vi "Controller VI.vi"(6 "Current Time In":u32, 7 "Read String":string, 8 "Down Detect Time In":u32, 9 "Up Detect Time In":u32, 10 "Left Detect Time In":u32, 11 "Right Detect Time In":u32) -> (0 "Down Detect Time Out":u32, 1 "Up Detect Time Out":u32, 2 "Left Detect Time Out":u32, 3 "Right detect Time Out":u32, 4 "Control Cluster":T1 {"Yaw Speed" scale=-1.0..1.0; "Vertical Speed" scale=-1.0..1.0; "Pitch" scale=-1.0..1.0; "Roll" scale=-1.0..1.0}, 5 "Command string":string)   [LabVIEW 2014]
uses:
  Others/Control cluster.ctl
  Global.vi
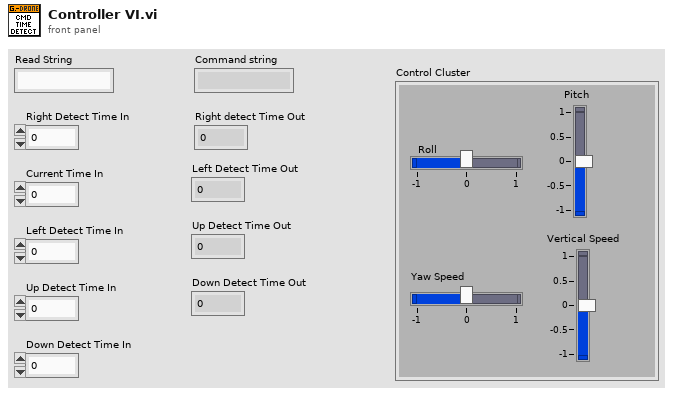
[diagram p1: front panel]
types:
  T1 = typedef "Control cluster.ctl" = cluster{"Roll":sgl, "Pitch":sgl, "Vertical Speed":sgl, "Yaw Speed":sgl}
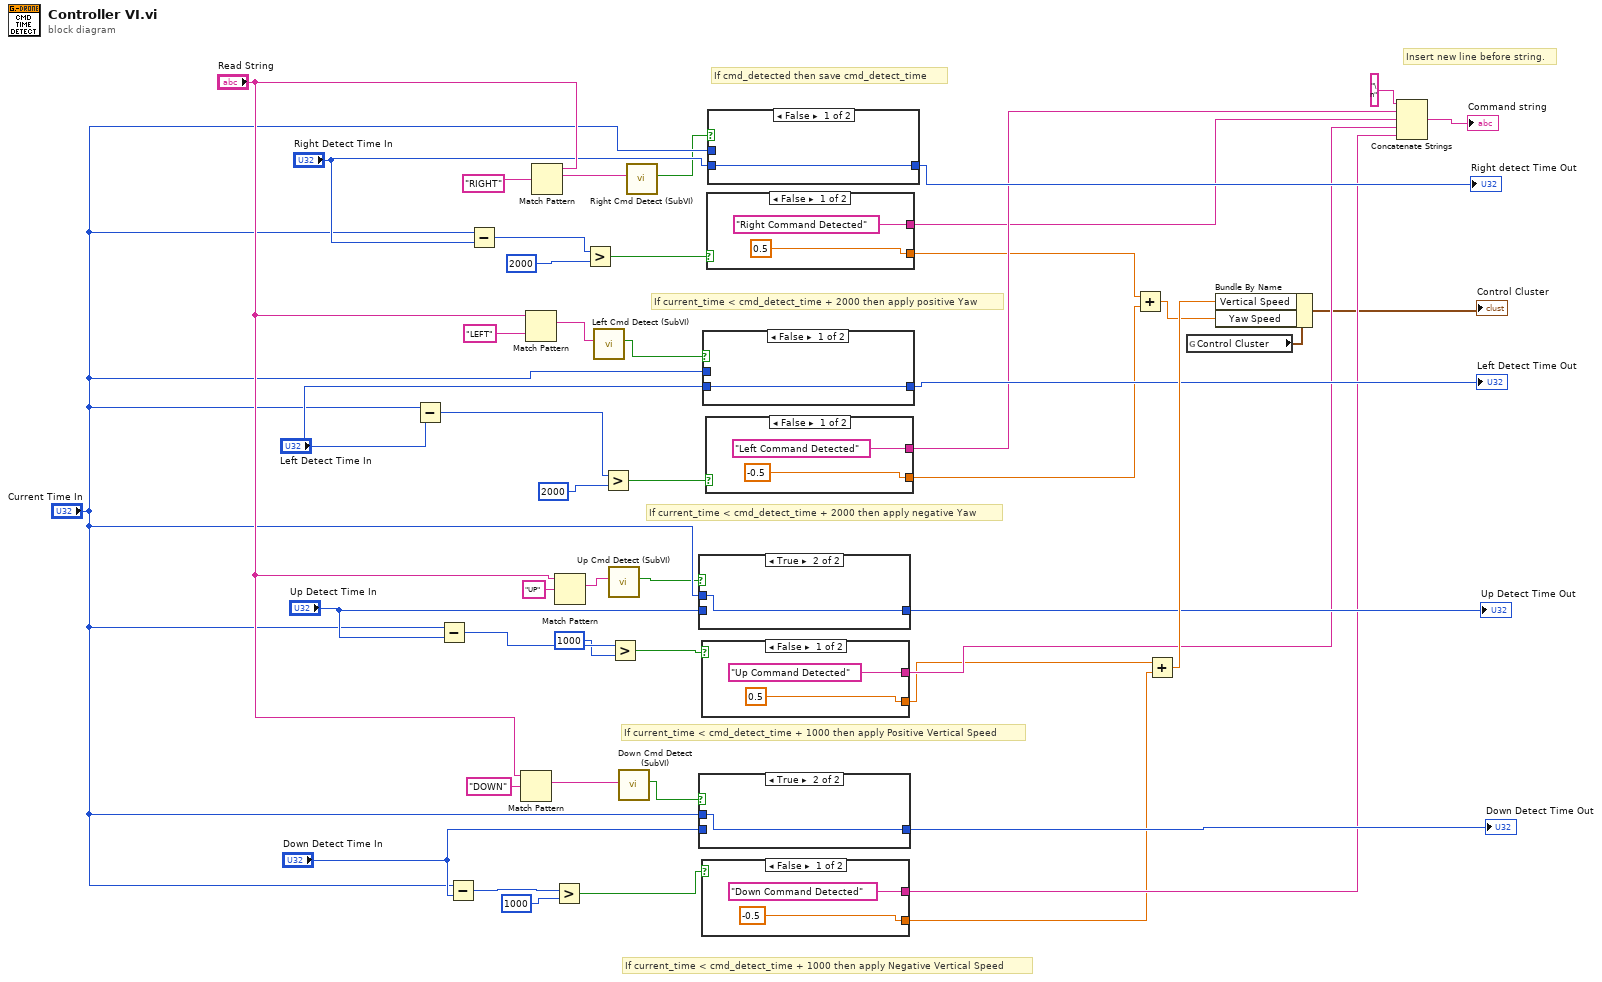
[diagram p0: block diagram]
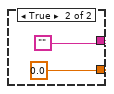
[diagram p2: hidden frame]
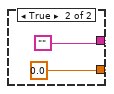
[diagram p4: hidden frame]
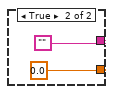
[diagram p6: hidden frame]
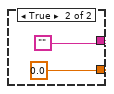
[diagram p8: hidden frame]
diagram:
  # "Insert new line before string."
  # "If current_time < cmd_detect_time + 1000 then apply Negative Vertical Speed"
  # "If current_time < cmd_detect_time + 1000 then apply Positive Vertical Speed"
  # "If current_time < cmd_detect_time + 2000 then apply negative Yaw"
  # "If cmd_detected then save cmd_detect_time"
  # "If current_time < cmd_detect_time + 2000 then apply positive Yaw"
  n1 = Subtract(x="Current Time In", y="Left Detect Time In") -> (x-y=w12:u32)
  n2 = Subtract(x="Current Time In", y="Up Detect Time In") -> (x-y=w20:u32)
  n3 = Subtract(x="Current Time In", y="Down Detect Time In") -> (x-y=w28:u32)
  n4 = Subtract(x="Current Time In", y="Right Detect Time In") -> (x-y=w4:u32)
  n5 = Match Pattern(string="Read String", regular expression="DOWN") -> (match substring=w32:string)  [unwired: 1 in, 3 out]
  n6 = Match Pattern(string="Read String", regular expression="LEFT") -> (match substring=w9:string)  [unwired: 1 in, 3 out]
  n7 = Match Pattern(string="Read String", regular expression="RIGHT") -> (match substring=w18:string)  [unwired: 1 in, 3 out]
  n8 = Greater?(x=w28, y=u32 1000) -> (0:w30:bool)
  n9 = Match Pattern(string="Read String", regular expression="UP") -> (match substring=w22:string)  [unwired: 1 in, 3 out]
  n10 = Greater?(x=w4, y=u32 2000) -> (0:w3:bool)
  n11 = call "Left Cmd Detect (SubVI).vi"("Read String"=w9) -> ("Left Command"=w10:bool)  [unwired: 10 in]
  n12 = Greater?(x=w12, y=u32 2000) -> (0:w13:bool)
  n13 = call "Up Cmd Detect (SubVI).vi"("Read String"=w22) -> ("Up Command"=w23:bool)  [unwired: 10 in]
  n14 = Greater?(x=w20, y=u32 1000) -> (0:w21:bool)
  n15 = call "Down Cmd Detect (SubVI).vi"("Read String"=w32) -> ("Down Command"=w31:bool)  [unwired: 10 in]
  n16 = call "Right Cmd Detect (SubVI).vi"("Read String"=w18) -> ("Right Command"=w17:bool)  [unwired: 10 in]
  n17 = case shown="True" w23 {
    tunnel: [w49 w50] -> w43
    tunnel: "Up Detect Time In" -> [w49 _]
    tunnel: "Current Time In" -> [_ w50]
    frame False {
    }
    frame True {
    }
  }
  "Up Detect Time Out" <- w43
  n18 = case shown="True" w31 {
    tunnel: [w51 w52] -> w38
    tunnel: "Down Detect Time In" -> [w51 _]
    tunnel: "Current Time In" -> [_ w52]
    frame False {
    }
    frame True {
    }
  }
  "Down Detect Time Out" <- w38
  n19 = case shown="False" w21 {
    tunnel: ["Up Command Detected" ""] -> w35
    tunnel: [0.5 0.0] -> w24
    frame False {
    }
    frame True {
    }
  }
  n20 = case shown="False" w30 {
    tunnel: ["Down Command Detected" ""] -> w34
    tunnel: [-0.5 0.0] -> w26
    frame False {
    }
    frame True {
    }
  }
  n21 = case shown="False" w10 {
    tunnel: [w61 w62] -> w42
    tunnel: "Left Detect Time In" -> [w61 _]
    tunnel: "Current Time In" -> [_ w62]
    frame False {
    }
    frame True {
    }
  }
  "Left Detect Time Out" <- w42
  n22 = case shown="False" w13 {
    tunnel: ["Left Command Detected" ""] -> w37
    tunnel: [-0.5 0.0] -> w15
    frame False {
    }
    frame True {
    }
  }
  n23 = case shown="False" w3 {
    tunnel: ["Right Command Detected" ""] -> w36
    tunnel: [0.5 0.0] -> w14
    frame False {
    }
    frame True {
    }
  }
  n24 = case shown="False" w17 {
    tunnel: [w71 w72] -> w44
    tunnel: "Right Detect Time In" -> [w71 _]
    tunnel: "Current Time In" -> [_ w72]
    frame False {
    }
    frame True {
    }
  }
  "Right detect Time Out" <- w44
  n25 = Add(x=w14, y=w15) -> (x+y=w16:dbl)
  n26 = Add(x=w24, y=w26) -> (x+y=w48:dbl)
  n27 = global read "Global.vi" "Control Cluster"() -> (w5:T1)
  n28 = Bundle By Name(cluster=w5, "Vertical Speed"=w48, "Yaw Speed"=w16) -> (→"Control Cluster":T1)
  n29 = Concatenate Strings("\n" ("string"), w37, w36, w35, w34) -> (→"Command string":string)
